vi "Sweep Load Currents.vi"(7 "Voltage values":dbl[](array[numeric]), 8 "error in":errorcluster, 11 "Measurement Configuration":T1={"Mode of operation"=enum."Perform measurement", "DUT setup time"=1.0, "Source delay"=0.005, "Aperture time"=0.005, "Nominal output voltage"=3.3, "Source resource name"="", "Source sense"=1009, "Source current limit"=25.0, "Source maximum power"=300.0, "Load resource name"="", "Load sense"=1009, "Load voltage limit range"=6.0, "Source Voltage"=6.0, "Load Current"=20.0} {"Load sense" items=["Local"=1008, "Remote"=1009]; "Source sense" items=["Local"=1008, "Remote"=1009]}) -> (0 "error out":errorcluster, 2 "Load sweep points":i32, 3 "Current values":dbl[](array[numeric]))   [LabVIEW 2021, in "Scalar Efficiency And Load Regulation_PMIC.lvlib"]
uses:
  Scalar Efficiency And Load Regulation_PMIC.lvlib
  Measurement Configuration.ctl
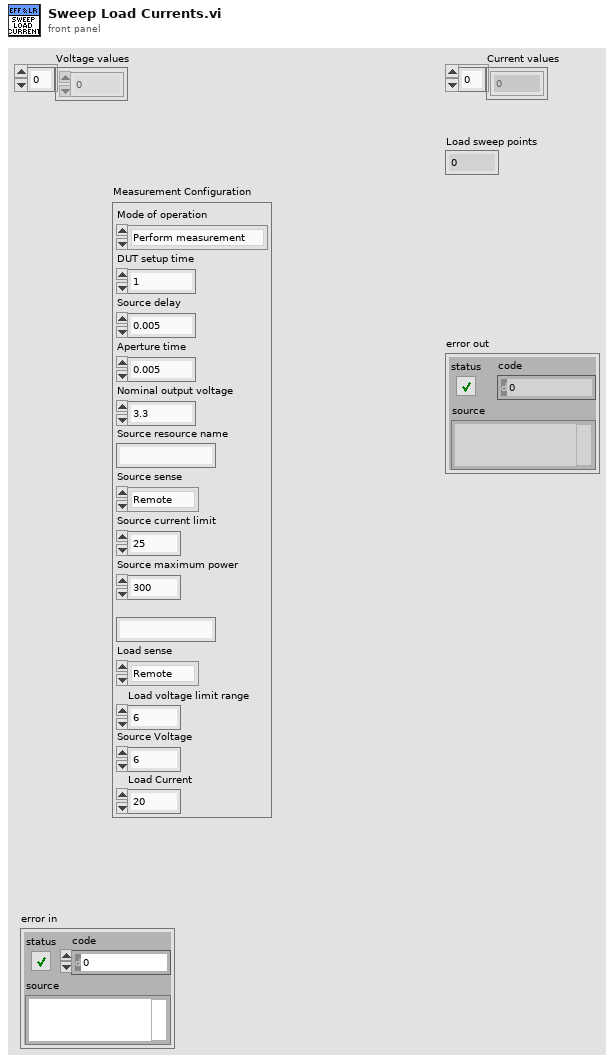
[diagram p1: front panel]
types:
  T1 = typedef "Scalar Efficiency And Load Regulation_PMIC.lvlib/Measurement Configuration.ctl" = cluster{"Mode of operation":enum32{"Power on the DUT", "Perform measurement", "Power off the DUT"}, "DUT setup time":dbl, "Source delay":dbl, "Aperture time":dbl, "Nominal output voltage":dbl, "Source resource name":string, "Source sense":i32, "Source current limit":dbl, "Source maximum power":dbl, "Load resource name":string, "Load sense":i32, "Load voltage limit range":dbl, "Source Voltage":dbl, "Load Current":dbl}
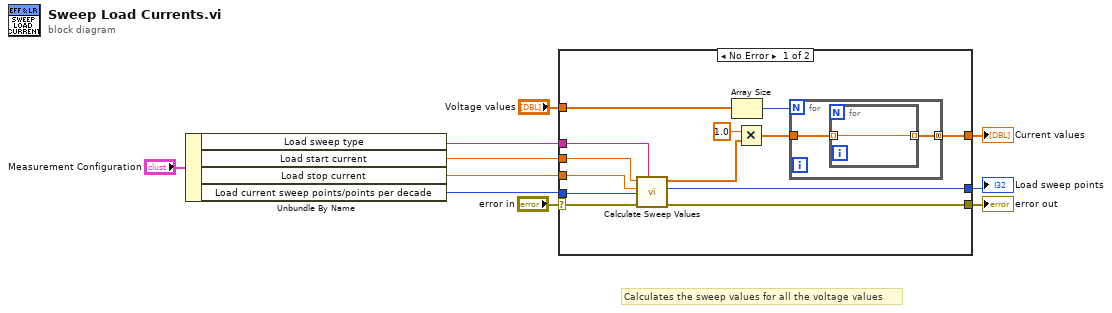
[diagram p0: block diagram]
diagram:
  # "Calculates the sweep values for all the voltage values"
  n1 = Unbundle By Name("Measurement Configuration") -> ("Load sweep type"=w6:string, "Load start current"=w5:dbl, "Load stop current"=w4:dbl, "Load current sweep points/points per decade"=w1:i32)
  n2 = case shown="No Error" "error in" {
    selector: "error in" -> [w14 w27]
    tunnel: w5 -> [w19 _]
    tunnel: w4 -> [w18 _]
    tunnel: w6 -> [w17 _]
    tunnel: [w22 _] -> w10
    tunnel: "Voltage values" -> [w20 _]
    tunnel: [w15 _] -> w9
    tunnel: [w13 w27] -> w7
    tunnel: w1 -> [w16 _]
    frame No Error {
      n3 = call "Calculate Sweep Values.vi"("Sweep type"=w17, "error in"=w14, "Points"=w16, "Stop level"=w18, "Start level"=w19) -> ("error out"=w13:errorcluster, "Sweep points"=w15:i32, "Sweep values"=w12:dbl[])  [unwired: 4 in]
      n4 = Array Size(array=w20) -> (size(s)=w23:i32)
      n5 = Multiply(x=1.0, y=w12) -> (x*y=w21:dbl[])
      n6 = for {
        N: w23 -> [_]
        tunnel: w21 -> [w25]
        tunnel: [w24] -> w22 mode=concatenating
        n7 = for {
          tunnel: w25 -> [w26] mode=indexing
          tunnel: [w26] -> w24 mode=indexing
        }
      }
    }
    frame Error {
    }
  }
  "Current values" <- w10
  "Load sweep points" <- w9
  "error out" <- w7
